vi "renderPopularVideos.vi"(8 "error in (no error)":errorcluster, 11 "YoutuberDownloader in":refnum<class "YoutuberDownloader.lvclass">) -> (0 "error out":errorcluster, 3 "YoutuberDownloader out":refnum<class "YoutuberDownloader.lvclass">)   [LabVIEW 2017, in "YoutuberDownloader.lvclass"]
uses:
  YoutuberDownloader.lvclass
  ConsoleOut/Print Options.ctl
  YoutuberDownloader.lvclass/YoutuberDownloader.ctl
  Video Class/Video.lvclass/Video.ctl
  ThirdPartyYoutubeLib Class/ThirdPartyYoutubeLib.lvclass
  Video Class/Video.lvclass
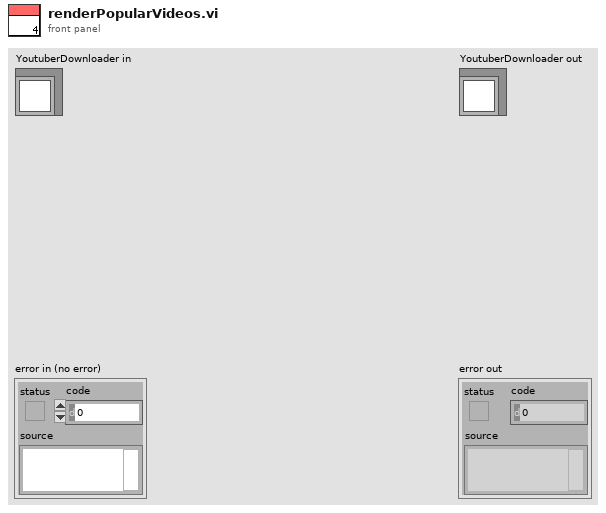
[diagram p1: front panel]
types:
  T1 = typedef "Print Options.ctl" = enum16{"Create", "Get Reference", "Print", "Print Header", "Close"}
  T2 = typedef "HashMap.ctl" = cluster{"Video Ids":string[], "Videos":refnum<class "Video.lvclass">[]}
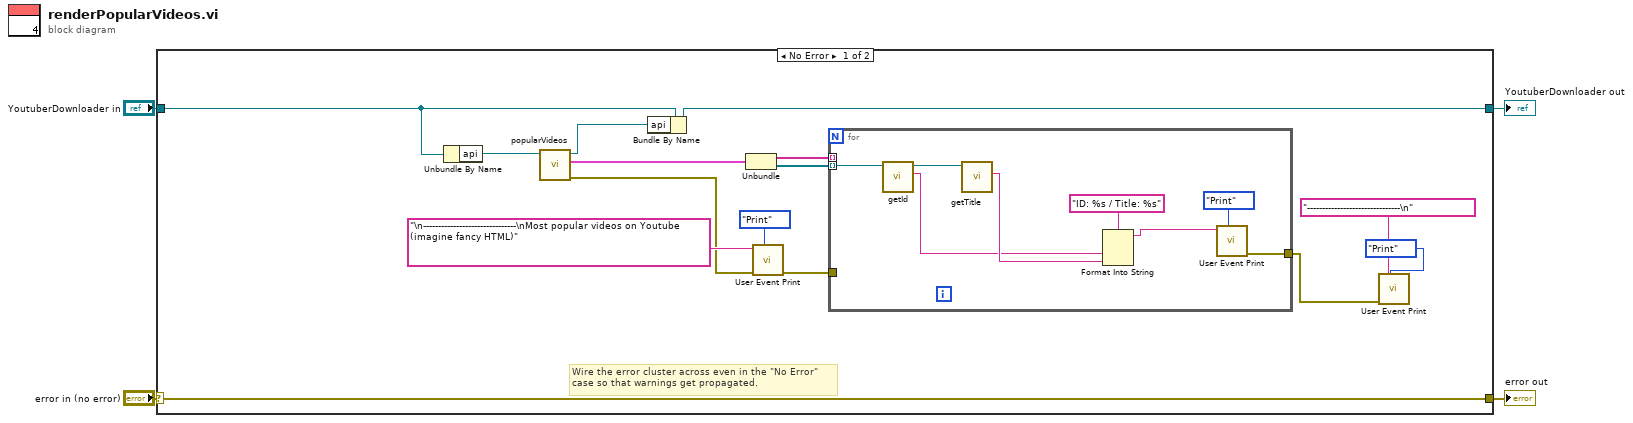
[diagram p0: block diagram]
diagram:
  n1 = case shown="No Error" "error in (no error)" {
    selector: "error in (no error)" -> [w19 w29]
    tunnel: [w19 w29] -> w3
    tunnel: [w6 w28] -> w1
    tunnel: "YoutuberDownloader in" -> [w18 w28]
    frame No Error {
      # "Wire the error cluster across even in the \"No Error\"\ncase so that warnings get propagated."
      n2 = Unbundle By Name(w18) -> ("api"=w17:refnum<class "ThirdPartyYoutubeLib.lvclass">)
      n3 = call-dynamic "popularVideos.vi"("ThirdPartyYoutubeLib in"=w17) -> ("error out"=w7:errorcluster, "HashMap"=w16:T2, "ThirdPartyYoutubeLib out"=w5:refnum<class "ThirdPartyYoutubeLib.lvclass">)  [unwired: 8 in]
      n4 = Bundle By Name(cluster=w18, "api"=w5) -> (w6:refnum<class "YoutuberDownloader.lvclass">)
      n5 = Unbundle(w16) -> ("Video Ids"=w15:string[], "Videos"=w14:refnum<class "Video.lvclass">[])
      n6 = call "User Event Print.vi"("Options"=Print_Options."Print", "error in (no error)"=w7, "String to Print"="\n-------------------------------\nMost popular videos on Youtube (imagine fancy HTML)" ("format string")) -> ("error out"=w11:errorcluster)  [unwired: 7 in, 1 out]
      n7 = for {
        tunnel: w15 -> [_] mode=indexing
        tunnel: w14 -> [w27] mode=indexing
        tunnel: w11 -> [_]
        tunnel: [w22] -> w10
        n8 = call "getId.vi"("Video in"=w27) -> ("id"=w20:string, "Video out"=w21:refnum<class "Video.lvclass">)  [unwired: 8 in, 1 out]
        n9 = call "getTitle.vi"("Video in"=w21) -> ("title"=w25:string)  [unwired: 8 in, 2 out]
        n10 = Format Into String(format string="ID: %s / Title: %s", w20, w25) -> (resulting string=w23:string)  [unwired: 2 in, 1 out]
        n11 = call "User Event Print.vi"("Options"=Print_Options."Print", "String to Print"=w23) -> ("error out"=w22:errorcluster)  [unwired: 8 in, 1 out]
      }
      n12 = call "User Event Print.vi"("Options"=Print_Options."Print", "error in (no error)"=w10, "String to Print"="-------------------------------\n") -> ()  [unwired: 7 in, 2 out]
    }
    frame Error {
    }
  }
  "error out" <- w3
  "YoutuberDownloader out" <- w1
